vi "Move_no_response.vi"(2 "Pulse Number":u32=100 min=1 max=500000, 4 "Axis Number":u8(ring)=1 items=["", "1", "2", "3", "4"], 5 "Port Number":i8=7 min=0) -> (1 "String Received":string)   [LabVIEW 2013]
panel:
  out "Command String":string
  # "Port Number 0=COM1"
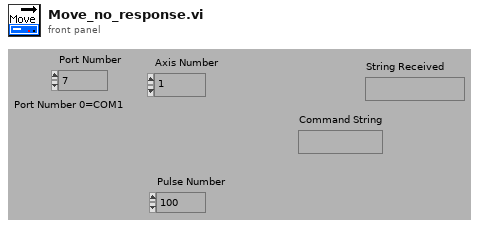
[diagram p1: front panel]
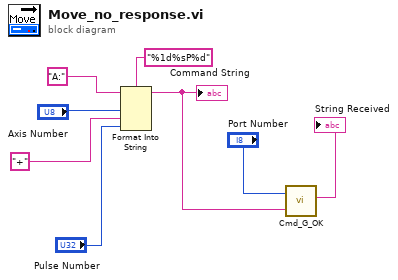
[diagram p0: block diagram]
diagram:
  n1 = Format Into String(format string="%1d%sP%d", initial string="A:", "Axis Number", "+", "Pulse Number") -> (resulting string=w4:string)  [unwired: 1 in, 1 out]
  "Command String" <- w4
  n2 = call "Cmd_G_OK.vi"("PortNumber"="Port Number", "Command String"=w4) -> ("Received String2"=→"String Received":string)  [unwired: 3 out]
